vi "Aula 21_09 Estruturas.vi"() -> ()   [LabVIEW 2020]
panel:
  out "Saída 3":dbl
  in  "Enum":T1(ring)
  out "Saída 2":dbl
  in  "Menu Ring":u16(ring) items=["TK para TC", "TF para TC", "TR para TC", "TF para TK"]
  in  "Text Ring":u16(ring) items=["TK para TC", "TF para TC", "TR para TC", "TF para TK", ""]
  out "Saída 1":dbl
  in  "Entrada":dbl
  in  "Stop Button":bool
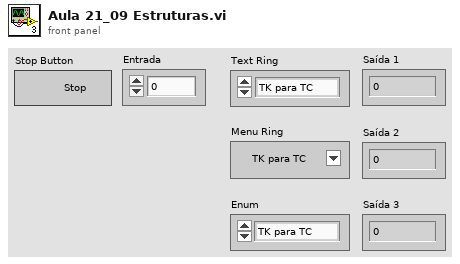
[diagram p1: front panel]
types:
  T1 = enum16{"TK para TC", "TF para TC", "TR para TC", "TF para TK", ""}
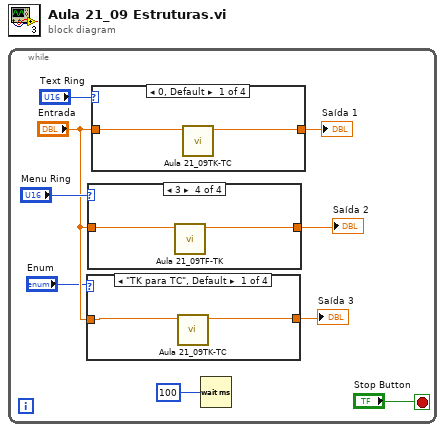
[diagram p0: block diagram]
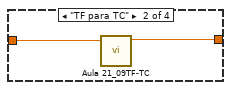
[diagram p2: hidden frame]
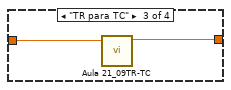
[diagram p3: hidden frame]
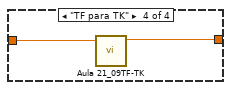
[diagram p4: hidden frame]
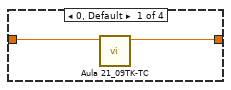
[diagram p5: hidden frame]
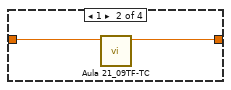
[diagram p6: hidden frame]
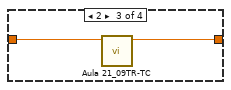
[diagram p7: hidden frame]
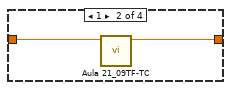
[diagram p8: hidden frame]
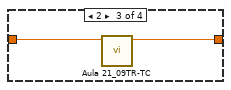
[diagram p9: hidden frame]
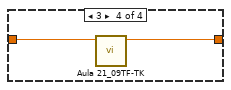
[diagram p10: hidden frame]
diagram:
  n1 = while {
    stop <- "Stop Button" stop-if-true
    n2 = case shown="\"TK para TC\", Default" "Enum" {
      tunnel: [w11 w13 w15 w17] -> w3
      tunnel: "Entrada" -> [w10 w12 w14 w16]
      frame "TK para TC", Default {
        n3 = call "Aula 21_09TK-TC.vi"("TK"=w10) -> ("TC"=w11:dbl)  [unwired: 10 in]
      }
      frame "TF para TC" {
        n4 = call "Aula 21_09TF-TC.vi"("TF"=w12) -> ("TC"=w13:dbl)  [unwired: 10 in]
      }
      frame "TR para TC" {
        n5 = call "Aula 21_09TR-TC.vi"("TR"=w14) -> ("TC"=w15:dbl)  [unwired: 10 in]
      }
      frame "TF para TK" {
        n6 = call "Aula 21_09TF-TK.vi"("TF"=w16) -> ("TK"=w17:dbl)  [unwired: 10 in]
      }
    }
    "Saída 3" <- w3
    n7 = case shown="3" "Menu Ring" {
      tunnel: "Entrada" -> [w19 w21 w23 w25]
      tunnel: [w18 w20 w22 w24] -> w4
      frame 0, Default {
        n8 = call "Aula 21_09TK-TC.vi"("TK"=w19) -> ("TC"=w18:dbl)  [unwired: 10 in]
      }
      frame 1 {
        n9 = call "Aula 21_09TF-TC.vi"("TF"=w21) -> ("TC"=w20:dbl)  [unwired: 10 in]
      }
      frame 2 {
        n10 = call "Aula 21_09TR-TC.vi"("TR"=w23) -> ("TC"=w22:dbl)  [unwired: 10 in]
      }
      frame 3 {
        n11 = call "Aula 21_09TF-TK.vi"("TF"=w25) -> ("TK"=w24:dbl)  [unwired: 10 in]
      }
    }
    "Saída 2" <- w4
    n12 = case shown="0, Default" "Text Ring" {
      tunnel: "Entrada" -> [w27 w29 w31 w33]
      tunnel: [w26 w28 w30 w32] -> w6
      frame 0, Default {
        n13 = call "Aula 21_09TK-TC.vi"("TK"=w27) -> ("TC"=w26:dbl)  [unwired: 10 in]
      }
      frame 1 {
        n14 = call "Aula 21_09TF-TC.vi"("TF"=w29) -> ("TC"=w28:dbl)  [unwired: 10 in]
      }
      frame 2 {
        n15 = call "Aula 21_09TR-TC.vi"("TR"=w31) -> ("TC"=w30:dbl)  [unwired: 10 in]
      }
      frame 3 {
        n16 = call "Aula 21_09TF-TK.vi"("TF"=w33) -> ("TK"=w32:dbl)  [unwired: 10 in]
      }
    }
    "Saída 1" <- w6
    n17 = Wait (ms)(milliseconds to wait=u32 100 ("millisecond timer value")) -> ()  [unwired: 1 out]
  }
